vi "S2C_Access_IncRow.vi"(8 "Error In":errorcluster, 11 "Coords":T1) -> (0 "Error Out":errorcluster)   [LabVIEW 2015]
doc: "Aquires front panel references, initializes the front panel, read all setting from the settings file, and reads all configurations from the config file."
uses:
  <vilib>/Utility/miscctls.llb/LVPoint32TypeDef.ctl
  S2C_Access_Globals.vi
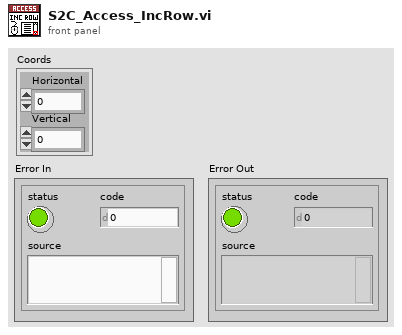
[diagram p1: front panel]
types:
  T1 = typedef "LVPoint32TypeDef.ctl" = cluster{"Horizontal":i32, "Vertical":i32}
  T2 = typedef "LVRowAndColumnUnsignedTypeDef.ctl" = cluster{"Row":u32, "Column":u32}
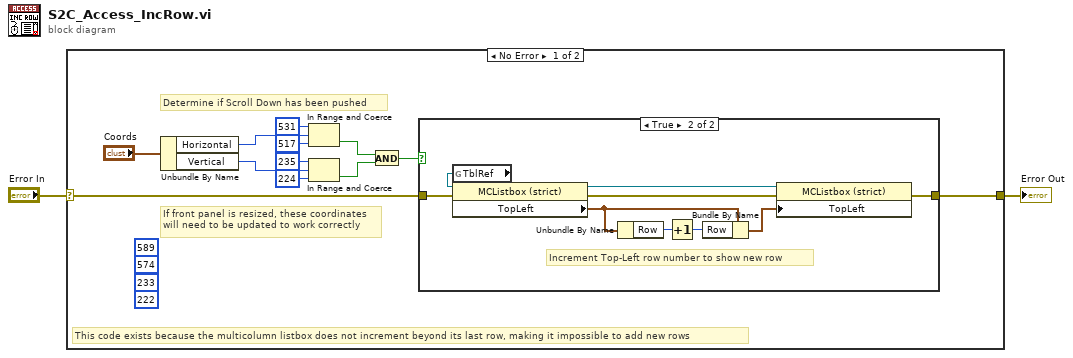
[diagram p0: block diagram]
diagram:
  n1 = case shown="No Error" "Error In" {
    selector: "Error In" -> [w3 w25]
    tunnel: [w4 w25] -> w2
    frame No Error {
      (unwired) 222 ("lower limit")
      (unwired) 233 ("upper limit")
      (unwired) 574 ("lower limit")
      (unwired) 589 ("upper limit")
      # "If front panel is resized, these coordinates\nwill need to be updated to work correctly"
      # "Determine if Scroll Down has been pushed"
      # "This code exists because the multicolumn listbox does not increment beyond its last row, making it impossible to add new rows"
      n2 = Unbundle By Name("Coords") -> ("Horizontal"=w7:i32, "Vertical"=w6:i32)
      n3 = In Range and Coerce(upper limit=531, x=w7, lower limit=517) -> (In Range?=w9:bool)  [unwired: 1 out]
      n4 = In Range and Coerce(upper limit=235, x=w6, lower limit=224) -> (In Range?=w10:bool)  [unwired: 1 out]
      n5 = And(x=w9, y=w10) -> (x .and. y?=w5:bool)
      n6 = case shown="True" w5 {
        tunnel: w3 -> [w15 w22]
        tunnel: [w15 w18] -> w4
        frame False {
          # "Not in range of listbox down arrow"
        }
        frame True {
          # "Increment Top-Left row number to show new row"
          n7 = global read "S2C_Access_Globals.vi" "TblRef"() -> (w16:refnum<vi>)
          n8 = property on="Property Node" class="MCListbox (strict)"(reference=w16, error in=w22) -> (reference out=w17:refnum<vi>, error out=w21:errorcluster, "TopLeft"=w19:T2)
          n9 = Unbundle By Name(w19) -> ("Row"=w24:u32)
          n10 = Increment(x=w24) -> (x+1=w23:u32)
          n11 = Bundle By Name(cluster=w19, "Row"=w23) -> (w20:T2)
          n12 = property on="Property Node" class="MCListbox (strict)"(reference=w17, error in=w21, "TopLeft"=w20) -> (error out=w18:errorcluster)  [unwired: 1 out]
        }
      }
    }
    frame Error {
    }
  }
  "Error Out" <- w2
